vi "SeCrTs-DI_Read.vi"(8 "error in (no error)":errorcluster, 9 "number of samples per channel":i32, 10 "DI_Task":refnum<k21>, 11 "Data FIFO Ref":T1) -> (0 "error out":errorcluster, 2 "task out":refnum<k21>)   [LabVIEW 2022 SP3]
uses:
  RT Controls/SeCrTs-Data FIFO.ctl
  <vilib>/Platform/TimedLoop/XDataNode/timing_clust.ctl
  <vilib>/Platform/TimedLoop/XDataNode/nitl_modes.ctl
  <vilib>/Platform/TimedLoop/XDataNode/wakeup.ctl
  RT Controls/SeCrTs-FGV Read write.ctl
  <vilib>/DAQmx/read.llb/DAQmx Read (Digital 1D Wfm NChan NSamp).vi
  <vilib>/DAQmx/miscellaneous.llb/DAQmx Fill In Error Info.vi
  <vilib>/Waveform/DTblOps.llb/DTbl Digital to Boolean Array.vi
  <vilib>/platform/TimedLoop/XDataNode/XDataNode.xnode
  <vilib>/Platform/TimedLoop/XDataNode/XDNodeRunTimeDep.lvlib
panel:
  out "# elements in queue":i32
  out "# pending remove":i32
  out "overflow? 2":bool
  out "overflow?":bool
  out "x-y":u32
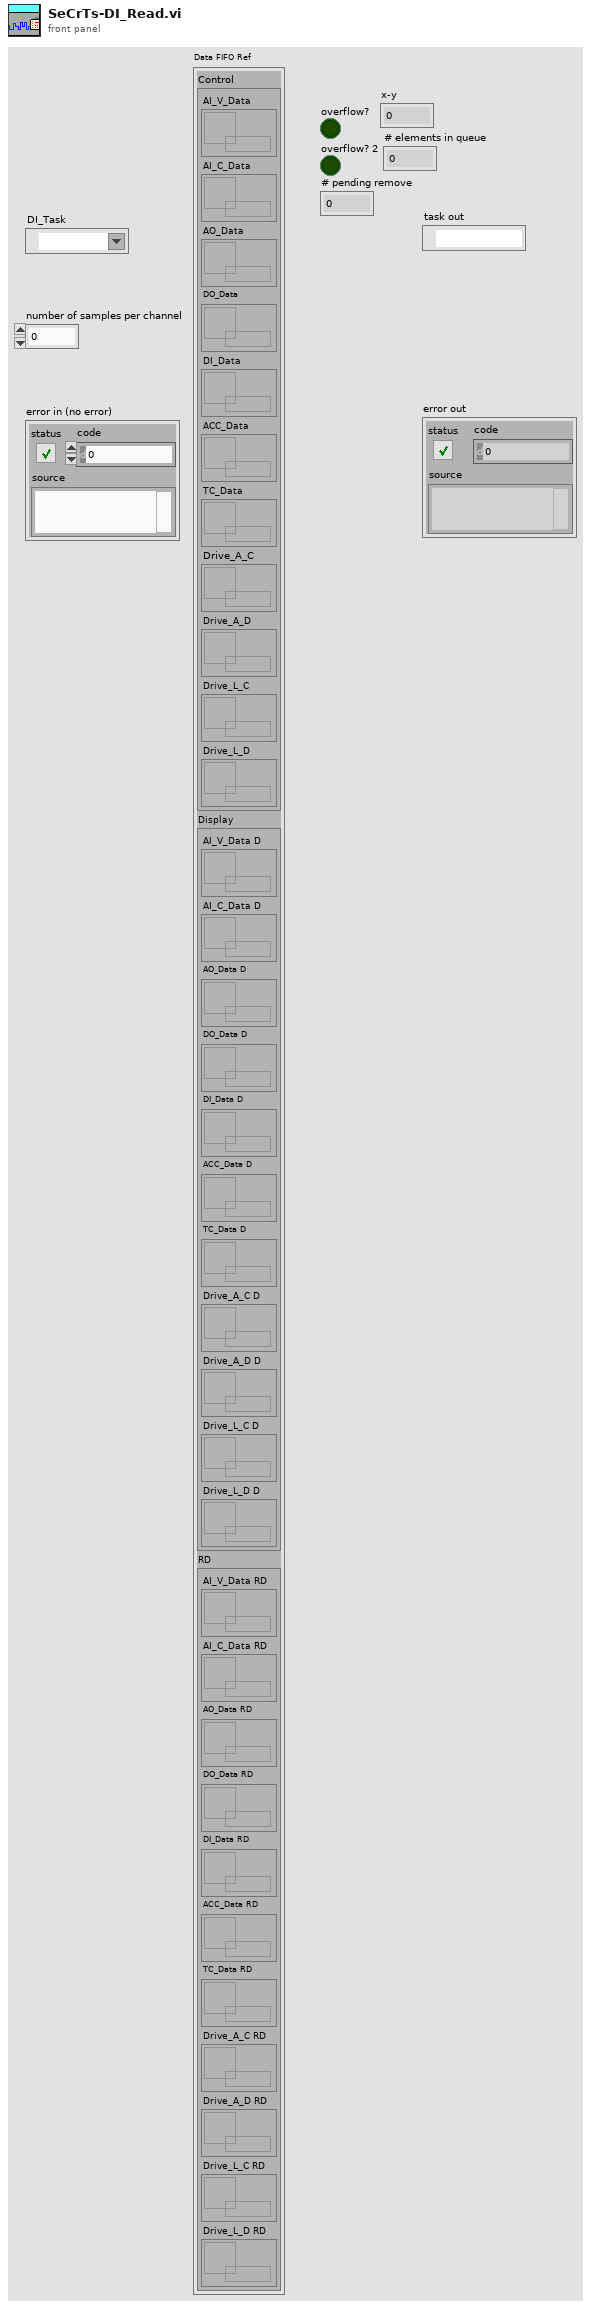
[diagram p1: front panel]
types:
  T1 = typedef "SeCrTs-Data FIFO.ctl" = cluster{"Control":cluster{"AI_V_Data":refnum<queue>, "AI_C_Data":refnum<queue>, "AO_Data":refnum<queue>, "DO_Data":refnum<queue>, "DI_Data":refnum<queue>, "ACC_Data":refnum<queue>, "TC_Data":refnum<queue>, "Drive_A_C":refnum<queue>, "Drive_A_D":refnum<queue>, "Drive_L_C":refnum<queue>, "Drive_L_D":refnum<queue>}, "Display":cluster{"AI_V_Data D":refnum<queue>, "AI_C_Data D":refnum<queue>, "AO_Data D":refnum<queue>, "DO_Data D":refnum<queue>, "DI_Data D":refnum<queue>, "ACC_Data D":refnum<queue>, "TC_Data D":refnum<queue>, "Drive_A_C D":refnum<queue>, "Drive_A_D D":refnum<queue>, "Drive_L_C D":refnum<queue>, "Drive_L_D D":refnum<queue>}, "RD":cluster{"AI_V_Data RD":refnum<queue>, "AI_C_Data RD":refnum<queue>, "AO_Data RD":refnum<queue>, "DO_Data RD":refnum<queue>, "DI_Data RD":refnum<queue>, "ACC_Data RD":refnum<queue>, "TC_Data RD":refnum<queue>, "Drive_A_C RD":refnum<queue>, "Drive_A_D RD":refnum<queue>, "Drive_L_C RD":refnum<queue>, "Drive_L_D RD":refnum<queue>}}
  T2 = cluster{"AO config":cluster{"Channel_Name":string, "Channel_Number":string, "Default_Value":dbl, "Units":string}[], "AI config":cluster{"Channel_Name":string, "Channel_Number":string, "Pre_Scale_min":dbl, "Pre_Scale_max":dbl, "Sensor_min":dbl, "Sensor_max":dbl, "Units":string}[], "DI config":cluster{"Channel_Name":string, "Channel_Number":string, "Default_Value":bool, "DI invert?":bool}[], "DO config":cluster{"Channel_Name":string, "Channel_Number":string, "Default_Value":bool, "DO invert?":bool}[], "TC config":cluster{"Channel_Name":string, "Channel_Number":string, "Pre_Scale_min":dbl, "Pre_Scale_max":dbl, "units":i32, "thermocouple type":i32}[], "ACC config":cluster{"Channel_Name":string, "Channel_Number":string, "Pre_Scale_min":dbl, "Pre_Scale_max":dbl, "Terminal configuration":i32, "Sensitivity":dbl, "Sensitivity units":i32}[], "SG config":cluster{"Channel_Name":string, "Channel_Number":string, "Pre_Scale_min":dbl, "Pre_Scale_max":dbl}[], "Strain Gauge Settings":cluster{"poisson ratio":dbl, "nominal gage resistance":dbl, "gage factor":dbl}, "Bridge Settings":cluster{"voltage excitation value":dbl, "voltage excitation source":i32, "initial bridge voltage":dbl, "lead wire resistance":dbl, "strain configuration":i32}, "Sample Rate":cluster{"AI Sample Rate":dbl[], "AO Sample Rate":dbl[], "DI Sample Rate":dbl[], "TC Sample Rate":dbl[], "DO Sample Rate":dbl[], "SG Sample Rate":dbl[], "ACC Sample Rate":dbl[]}}
  T3 = cluster{"Channel_Name":string, "Channel_Number":string, "Default_Value":bool, "DI invert?":bool}[]
  T4 = typedef "XDNodeRunTimeDep.lvlib/timing_clust.ctl" = cluster{"Expected End [f-1]":u64, "Actual End [f-1]":u64, "Finished Late? [f-1]":bool, "Expected End [i-1]":u64, "Actual End [i-1]":u64, "Finished Late? [i-1]":bool, "Expected Start [i]":u64, "Actual Start [i]":u64, "Expected Start [f]":u64, "Actual Start [f]":u64, "Source Name":string, "Structure Name":string, "Period":i64, "Deadline":i64, "Offset":i64, "Start":i64, "Priority":i32, "Timeout":i32, "Mode":T5, "Wakeup Reason":T6, "Error":errorcluster, "Source Type":string, "Secondary Source Type":string, "Global End Time":u64, "Global Start Time":u64, "Frame Duration":u64, "Iteration Duration":u64, "Assigned CPU":i32, "I/O Scan Engine Mode":u32}
  T5 = typedef "XDNodeRunTimeDep.lvlib/nitl_modes.ctl" = enum32{"No Change", "Process missed periods, maintain original phase", "Discard missed periods, maintain original phase", "Process missed periods, ignore original phase", "Discard missed periods, ignore original phase"}
  T6 = typedef "XDNodeRunTimeDep.lvlib/wakeup.ctl" = enum32{"Normal", "Aborted", "Asynchronous wakeup", "Timing source error", "Timed loop error", "Timeout"}
  T7 = typedef "SeCrTs-FGV Read write.ctl" = enum16{"Write", "Read"}
  T8 = enum16{"AI C", "AI V", "AO", "DI", "DO", "TC", "ACC", "DR L", "DR A"}
  T9 = enum16{"Init", "Read 'All'", "Read 'n'", "Read '1'", "Write '1'", "Write 'n'", "Write 'All'"}
  T10 = cluster{"Start DAQ":bool, "Stop DAQ":bool, "RT Stop":bool, "RT Exit":bool, "Start Seq":bool}
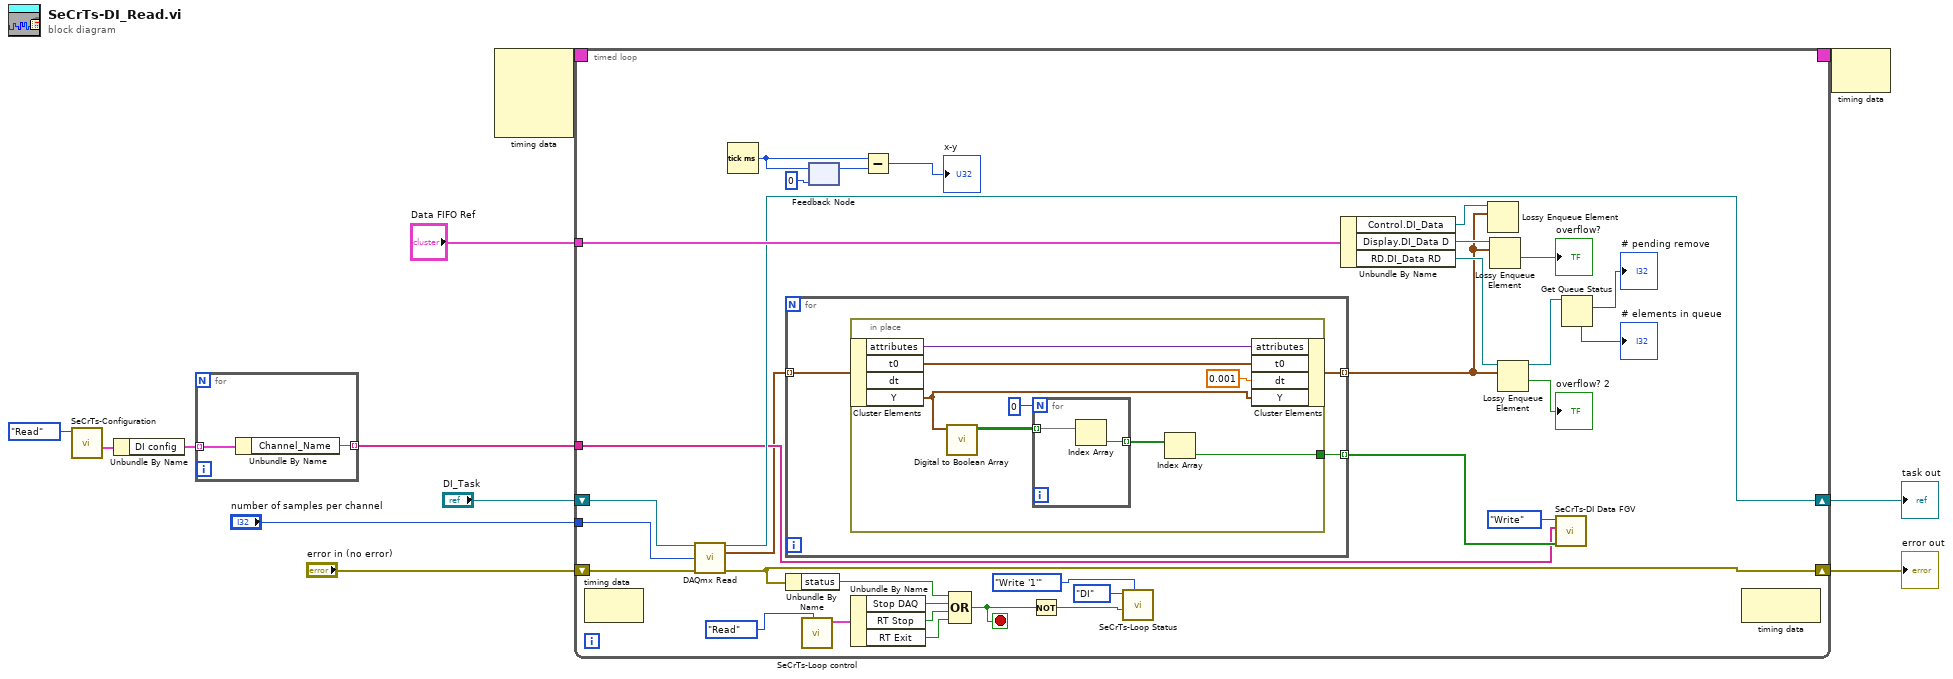
[diagram p0: block diagram]
diagram:
  n1 = call "SeCrTs-Configuration.vi"("Enum"=enum16{"Write", "Read"}."Read") -> ("Config out"=w5:T2)  [unwired: 10 in]
  n2 = Unbundle By Name(w5) -> ("DI config"=w4:T3)
  n3 = for {
    tunnel: w4 -> [w14] mode=indexing
    tunnel: [w13] -> w3 mode=indexing
    n4 = Unbundle By Name(w14) -> ("Channel_Name"=w13:string)
  }
  n5 = node-c288() -> (w2:T4)  [unwired: 4 in]
  n6 = timed-loop {
    tunnel: "number of samples per channel" -> [w31]
    tunnel: "Data FIFO Ref" -> [w30]
    shift-right: [w25] -> w8
    shift-left: "DI_Task" -> [w46]
    shift-right: [w24] -> w7
    shift-left: "error in (no error)" -> [w45]
    tunnel: w3 -> [w22]
    timing: w2 -> [_]
    timing-out: [_] -> w1
    stop <- w47 stop-if-true
    n7 = node-c288() -> ()  [unwired: 1 in, 1 out]
    n8 = call-poly <vilib>:"DAQmx Read.vi"("task/channels in"=w46, "number of samples per channel"=w31, "error in"=w45) -> ("task out"=w25:refnum<k21>, "data"=w16:digitalwaveform[], "error out"=w24:errorcluster)  [unwired: 10 in]
    n9 = Tick Count (ms)() -> (millisecond timer value=w35:u32)
    n10 = for {
      tunnel: w16 -> [w51] mode=indexing
      tunnel: [w52] -> w23 mode=indexing
      tunnel: [w50] -> w15 mode=indexing
      n11 = in-place {
        in-place-border: [w57] -> w52
        n12 = in-place-cluster #1(w51) -> ("attributes"=w53:variant, "t0"=w54:timestamp, "Y"=w56:digitaldata)  [unwired: 1 out]
        n13 = call-poly <vilib>:"Digital to Boolean Array.vi"("digital data"=w56) -> ("boolean array"=w59:bool[][])  [unwired: 9 in, 1 out]
        n14 = for {
          N: 0 -> [_]
          tunnel: w59 -> [w62] mode=indexing
          tunnel: [w61] -> w58 mode=indexing
          n15 = Index Array(array=w62) -> (element=w61:bool)  [unwired: 1 in]
        }
        n16 = Index Array(array=w58) -> (element=w57:bool)  [unwired: 1 in]
        n17 = in-place-cluster #1("attributes"=w53, "t0"=w54, "dt"=0.001, "Y"=w56) -> (w50:digitalwaveform)
      }
    }
    n18 = Unbundle By Name(w24) -> ("status"=w44:bool)
    n19 = call "SeCrTs-Loop control.vi"("Action"=enum16{"Init", "Write", "Read"}."Read") -> ("Loop Control out"=w39:T10)  [unwired: 9 in, 1 out]
    n20 = feedback-in #2(w35) -> ()
    n21 = feedback #2(u32 0 ("millisecond timer value")) -> (w34:u32)
    n22 = Unbundle By Name(w39) -> ("Stop DAQ"=w43:bool, "RT Stop"=w42:bool, "RT Exit"=w41:bool)
    n23 = Subtract(x=w35, y=w34) -> (x-y=→"x-y":u32)
    n24 = Compound Arithmetic op=OR(w44, w43, w42, w41) -> (w47:bool)
    n25 = Not(x=w47) -> (.not. x?=w36:bool)
    n26 = call "SeCrTs-Loop Status.vi"("Option"=T9."Write '1'", "Status"=w36, "Loop"=T8."DI") -> ()  [unwired: 6 in, 3 out]
    n27 = Unbundle By Name(w30) -> ("Control.DI_Data"=w29:refnum<queue>, "Display.DI_Data D"=w28:refnum<queue>, "RD.DI_Data RD"=w27:refnum<queue>)
    n28 = Lossy Enqueue Element(queue=w29, element=w15) -> ()  [unwired: 1 in, 4 out]
    n29 = Lossy Enqueue Element(queue=w28, element=w15) -> (overflow?=→"overflow?":bool)  [unwired: 1 in, 3 out]
    n30 = Lossy Enqueue Element(queue=w27, element=w15) -> (queue out=w19:refnum<queue>, overflow?=→"overflow? 2":bool)  [unwired: 1 in, 2 out]
    n31 = call "SeCrTs-DI Data FGV.vi"("DI Y LP"=w23, "DI Signal List LP"=w22, "Write/Read"=SeCrTs-FGV_Read_write."Write") -> ()  [unwired: 6 in, 3 out]
    n32 = Get Queue Status(queue=w19) -> (# pending remove=→"# pending remove":i32, # elements in queue=→"# elements in queue":i32)  [unwired: 2 in, 6 out]
    n33 = node-c288() -> ()  [unwired: 1 in, 1 out]
  }
  "task out" <- w8
  "error out" <- w7
  n34 = node-c288(w1) -> ()  [unwired: 1 out]
